vi "linear interp iiii- complex - z-omega.vi"(0 "z":cdb[](array[numeric]), 5 "omega":dbl[](array[numeric]), 11 "center":i32=-1) -> (2 "directed sigma":cdb, 3 "directed sigma - abs":dbl, 4 "z out":cdb[](array[numeric]), 6 "omega out":dbl[](array[numeric]), 8 "left":cdb, 10 "center":cdb, 12 "intercept":cdb, 13 "slope":cdb, 15 "right":cdb)   [LabVIEW 2018]
uses:
  <vilib>/Analysis/NI_AALBase.lvlib
  <vilib>/Analysis/baseanly.llb/Complex A x B.vi
  <vilib>/Analysis/Matrix/NI_Matrix.lvlib
  <vilib>/Analysis/Matrix/Numeric/Conversions/Array To Matrix - RA2.vi
  <vilib>/Analysis/baseanly.llb/Real Inverse Matrix.vi
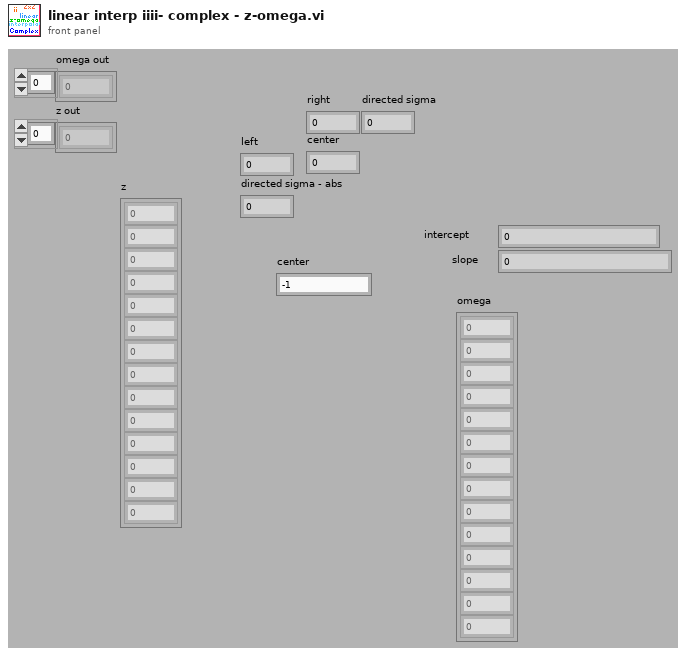
[diagram p1: front panel]
types:
  T1 = typedef "NI_Matrix.lvlib/RealMatrix.ctl" = dbl[][]
  T2 = typedef "NI_Matrix.lvlib/ComplexMatrix.ctl" = cdb[][]
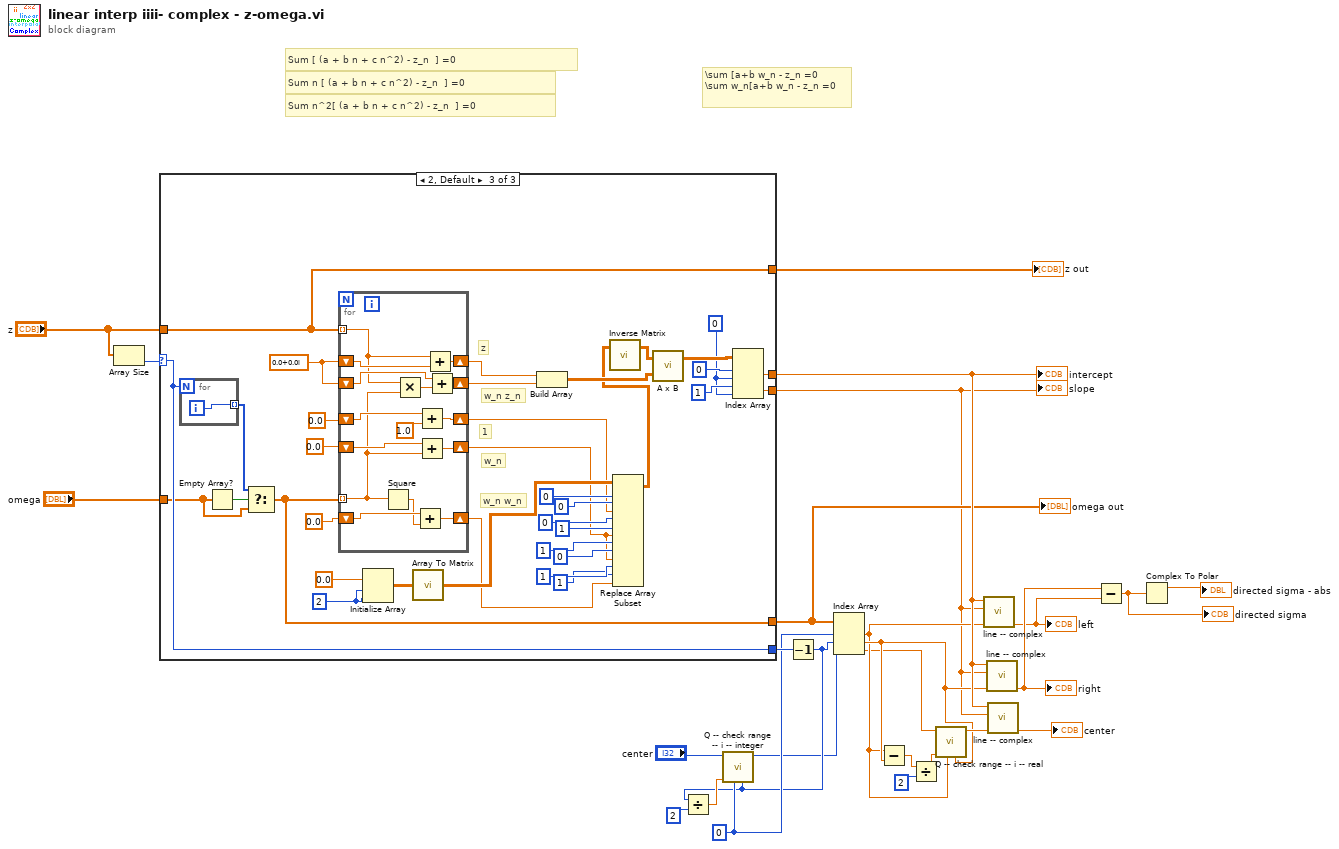
[diagram p0: block diagram]
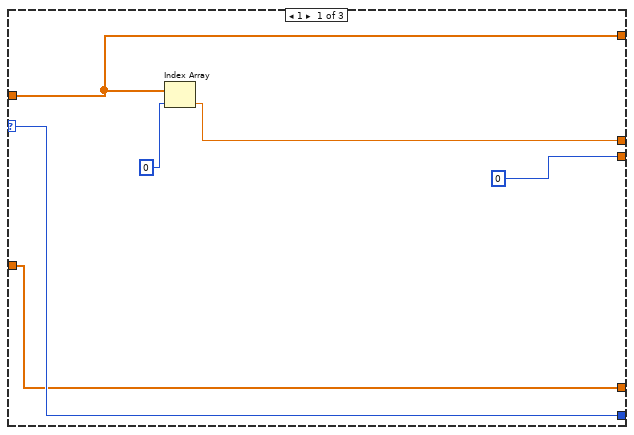
[diagram p2: hidden frame]
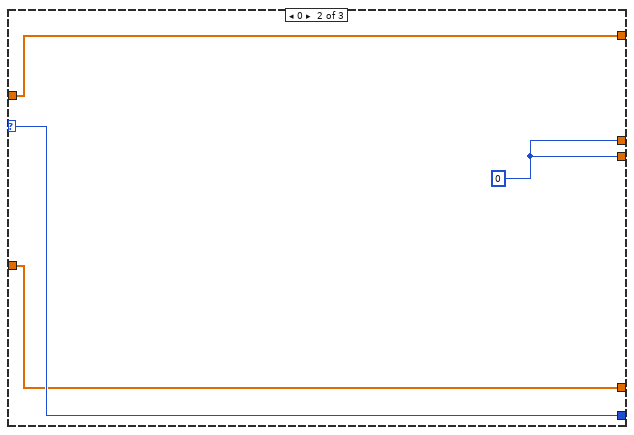
[diagram p3: hidden frame]
diagram:
  w3 = 0 ("n")
  # "\\sum [a+b w_n - z_n =0 \n\\sum w_n[a+b w_n - z_n =0"
  # "Sum n^2[ (a + b n + c n^2) - z_n  ] =0"
  # "Sum n [ (a + b n + c n^2) - z_n  ] =0"
  # "Sum [ (a + b n + c n^2) - z_n  ] =0"
  n1 = Array Size(array="z") -> (size(s)=w15:i32)
  n2 = case shown="2, Default" w15 {
    selector: w15 -> [w30 w36 w61]
    tunnel: [w31 w35 w63] -> w17
    tunnel: [0 ("index") w35 w62] -> w8
    tunnel: "z" -> [w27 w34 w37]
    tunnel: [w30 w36 w61] -> w20
    tunnel: "omega" -> [w28 w33 w59]
    tunnel: [w28 w33 w38] -> w13
    tunnel: [w27 w34 w37] -> w12
    frame 1 {
      n3 = Index Array(array=w27, index=0) -> (element=w31:cdb)
    }
    frame 0 {
      w35 = 0 ("index")
    }
    frame 2, Default {
      w57 = 2 ("n")
      w64 = 0 ("index (row)")
      w71 = cdb 0.0+0.0i
      # "w_n w_n"
      # "w_n"
      # "1"
      # "w_n z_n"
      # "z"
      n4 = for {
        N: w61 -> [_]
        tunnel: [w73] -> w58 mode=indexing
        i -> [w73]
      }
      n5 = Empty Array?(array=w59) -> (empty?=w60:bool)
      n6 = Select(t=w58, s=w60, f=w59) -> (s? t:f=w38:dbl[])
      n7 = for {
        tunnel: w37 -> [w83] mode=indexing
        shift-right: [w88] -> w70
        shift-left: w71 -> [w87]
        shift-right: [w85] -> w69
        shift-left: w71 -> [w84]
        shift-right: [w81] -> w47
        shift-left: 0.0 -> [w82]
        shift-right: [w78] -> w42
        shift-left: 0.0 -> [w79]
        tunnel: w38 -> [w75] mode=indexing
        shift-right: [w76] -> w41
        shift-left: 0.0 -> [w77]
        n8 = Square(x=w75) -> (x^2=w74:dbl)
        n9 = Multiply(x=w83, y=w75) -> (x*y=w86:cdb)
        n10 = Add(x=w77, y=w74) -> (x+y=w76:dbl)
        n11 = Add(x=w82, y=1.0) -> (x+y=w81:dbl)
        n12 = Add(x=w79, y=w75) -> (x+y=w78:dbl)
        n13 = Add(x=w83, y=w87) -> (x+y=w88:cdb)
        n14 = Add(x=w84, y=w86) -> (x+y=w85:cdb)
      }
      n15 = Initialize Array(0.0 ("n"), w57, w57) -> (w51:dbl[][])
      n16 = call-poly <vilib>:"Array To Matrix.vi"("Real 2D Array"=w51) -> ("Real Matrix"=w56:T1)
      n17 = Build Array(w70, w69) -> (w68:T2)
      n18 = Replace Array Subset(array=w56, new element #1=w47, index (row) #1=0 ("n"), index (col) #1=0 ("n"), new element #2=w42, index (row) #2=0 ("n"), index (col) #2=1 ("n"), new element #3=w42, index (row) #3=1 ("n"), index (col) #3=0 ("n"), new element #4=w41, index (row) #4=1 ("n"), index (col) #4=1 ("n")) -> (w40:T1)
      n19 = call-poly <vilib>:"Inverse Matrix.vi"("Input Matrix"=w40) -> ("Inverse Matrix"=w39:T1)  [unwired: 1 in, 1 out]
      n20 = call-poly <vilib>:"A x B.vi"("B"=w68, "A"=w39) -> ("A x B"=w67:T2)  [unwired: 1 out]
      n21 = Index Array(array=w67, index (row) #1=0 ("index (row)"), index (col) #1=w64, index (row) #2=1 ("index (row)"), index (col) #2=w64) -> (element #1=w63:cdb, element #2=w62:cdb)
    }
  }
  "slope" <- w8
  "intercept" <- w17
  "omega out" <- w13
  "z out" <- w12
  n22 = Decrement(x=w20) -> (x-1=w2:i32)
  n23 = Divide(x=w2, y=2 ("n")) -> (x/y=w5:dbl)
  n24 = call "Q -- check range -- i -- integer.vi"("upper"=w2, "lower"=w3, "default"=w5, "number"="center") -> ("number in range"=w1:i32)  [unwired: 5 in, 2 out]
  n25 = Index Array(array=w13, index #1=w3, index #2=w2, index #3=w1) -> (element #1=w10:dbl, element #2=w11:dbl, element #3=w7:dbl)
  n26 = Subtract(x=w10, y=w11) -> (x-y=w9:dbl)
  n27 = Divide(x=w9, y=2 ("n")) -> (x/y=w21:dbl)
  n28 = call "Q -- check range -- i -- real.vi"("upper"=w11, "lower"=w10, "default"=w21, "number"=w7) -> ("number in range"=w25:dbl)  [unwired: 5 in, 2 out]
  n29 = call "line -- complex.vi"("n"=w10, "slope"=w8, "intercept"=w17) -> ("value"=w22:cdb)  [unwired: 7 in, 1 out]
  "left" <- w22
  n30 = call "line -- complex.vi"("n"=w11, "slope"=w8, "intercept"=w17) -> ("value"=w23:cdb)  [unwired: 7 in, 1 out]
  "right" <- w23
  n31 = call "line -- complex.vi"("n"=w25, "slope"=w8, "intercept"=w17) -> ("value"=→"center":cdb)  [unwired: 7 in, 1 out]
  n32 = Subtract(x=w23, y=w22) -> (x-y=w18:cdb)
  "directed sigma" <- w18
  n33 = Complex To Polar(r * e^(i*theta)=w18) -> (r=→"directed sigma - abs":dbl)  [unwired: 1 out]
